vi "Get all TwinCAT variables.vi"() -> ()   [LabVIEW 2021]
uses:
  Program Files (x86)/Beckhoff/TwinCAT/Common64/TcAdsDll.dll
panel:
  out "Variables":T1(array[cluster])
  in  "AMS net ID":cluster{u8, u8, u8, u8, u8, u8}={5, 94, 0, 254, 1, 1}
  in  "Port":u16=851
  out "nSymSize":u32
  out "# symbols":u32
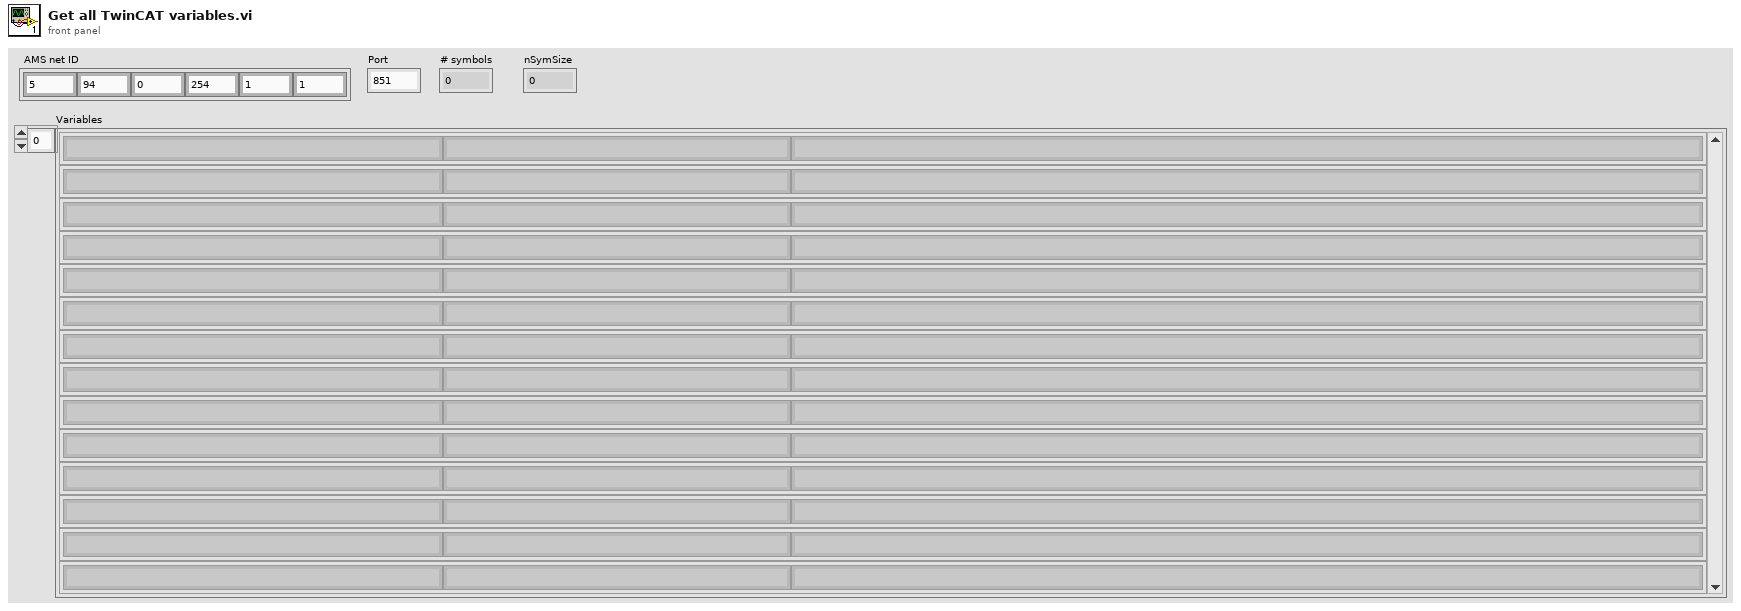
[diagram p1: front panel]
types:
  T1 = cluster{"Name":string, "Type":string, "Comment":string}[]
  T2 = cluster{"AMS net ID":cluster{u8, u8, u8, u8, u8, u8}, "Port":u16}
  T3 = enum16{"big-endian, network order", "native, host order", "little-endian"}
  T4 = cluster{"EntryLenght":u32, "iGroup":u32, "iOffset":u32, "iSize":u32, "DataType":u32, "Flags":u32, "nameLength":u16, "typeLength":u16, "commentLength":u16}
  T5 = cluster{"string":string, "string":string, "string":string}
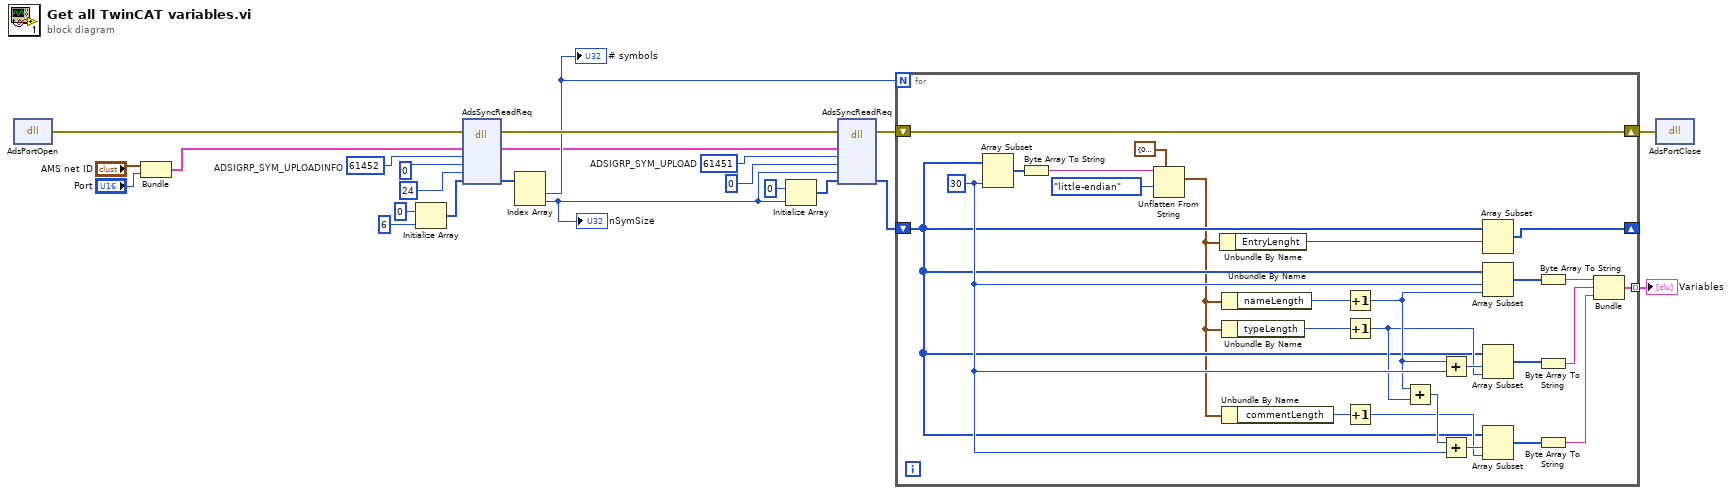
[diagram p0: block diagram]
diagram:
  w9 = 61451  # ADSIGRP_SYM_UPLOAD
  w20 = 61452  # ADSIGRP_SYM_UPLOADINFO
  n1 = dll-call lib="C:/Program Files (x86)/Beckhoff/TwinCAT/Common64/TcAdsDll.dll" fn="AdsPortOpen"() -> (error out=w21:errorcluster)  [unwired: 4 in, 1 out]
  n2 = Bundle("AMS net ID"="AMS net ID", "Port"="Port") -> (w3:T2)  [unwired: 1 in]
  n3 = Initialize Array(u32 0 ("dimension size"), 6 ("dimension size")) -> (w15:u32[])
  n4 = dll-call lib="C:/Program Files (x86)/Beckhoff/TwinCAT/Common64/TcAdsDll.dll" fn="AdsSyncReadReq"(error in=w21, "pAddr"=w3, "nIndexGroup"=w20, "nIndexOffset"=u32 0, "nLength"=u32 24, "pData"=w15) -> (error out=w13:errorcluster, "pData"=w14:u32[])  [unwired: 7 in, 1 out]
  n5 = Index Array(array=w14) -> (element #1=w6:u32, element #2=w10:u32)  [unwired: 2 in]
  "# symbols" <- w6
  "nSymSize" <- w10
  n6 = Initialize Array(u8 0 ("element"), w10) -> (w11:u8[])
  n7 = dll-call lib="C:/Program Files (x86)/Beckhoff/TwinCAT/Common64/TcAdsDll.dll" fn="AdsSyncReadReq"(error in=w13, "pAddr"=w3, "nIndexGroup"=w9, "nIndexOffset"=u32 0, "nLength"=w10, "pData"=w11) -> (error out=w4:errorcluster, "pData"=w7:u8[])  [unwired: 7 in, 1 out]
  n8 = for {
    N: w6 -> [_]
    shift-right: [w30] -> _
    shift-left: w7 -> [w31]
    shift-right: [w28] -> w2
    shift-left: w4 -> [w28]
    tunnel: [w23] -> w1 mode=indexing
    w41 = 30 ("length")
    n9 = Array Subset(array=w31, length=w41) -> (w46:u8[])  [unwired: 1 in]
    n10 = Byte Array To String(unsigned byte array=w46) -> (string=w48:string)
    n11 = Unflatten From String(type=T4 {"EntryLenght"=0, "iGroup"=0, "iOffset"=0, "iSize"=0, "DataType"=0, "Flags"=0, "nameLength"=0, "typeLength"=0, "commentLength"=0}, binary string=w48, byte order (0:big-endian, network order)=T3."little-endian") -> (value=w27:T4)  [unwired: 2 in, 2 out]
    n12 = Unbundle By Name(w27) -> ("EntryLenght"=w29:u32)
    n13 = Unbundle By Name(w27) -> ("nameLength"=w37:u16)
    n14 = Unbundle By Name(w27) -> ("typeLength"=w35:u16)
    n15 = Unbundle By Name(w27) -> ("commentLength"=w33:u16)
    n16 = Increment(x=w37) -> (x+1=w36:u16)
    n17 = Increment(x=w35) -> (x+1=w34:u16)
    n18 = Increment(x=w33) -> (x+1=w32:u16)
    n19 = Add(x=w36, y=w34) -> (x+y=w38:u16)
    n20 = Add(x=w36, y=w41) -> (x+y=w39:i32)
    n21 = Add(x=w38, y=w41) -> (x+y=w40:i32)
    n22 = Array Subset(array=w31, index=w29) -> (w30:u8[])  [unwired: 1 in]
    n23 = Array Subset(array=w31, index=w41, length=w36) -> (w44:u8[])
    n24 = Array Subset(array=w31, index=w39, length=w34) -> (w43:u8[])
    n25 = Array Subset(array=w31, index=w40, length=w32) -> (w42:u8[])
    n26 = Byte Array To String(unsigned byte array=w44) -> (string=w26:string)
    n27 = Byte Array To String(unsigned byte array=w43) -> (string=w25:string)
    n28 = Byte Array To String(unsigned byte array=w42) -> (string=w24:string)
    n29 = Bundle("string"=w26, "string"=w25, "string"=w24) -> (w23:T5)  [unwired: 1 in]
  }
  "Variables" <- w1
  n30 = dll-call lib="C:/Program Files (x86)/Beckhoff/TwinCAT/Common64/TcAdsDll.dll" fn="AdsPortClose"(error in=w2) -> ()  [unwired: 3 in, 2 out]
